vi "Read PinLevels.vi"(11 "niDigital in":refnum<class "niDigital.lvclass">) -> (2 "PinLevels":string="C:\\Sandbox\\Supporting Materials\\Digital\\Levels\\levelsheet.digilevels", 3 "niDigital out":refnum<class "niDigital.lvclass">)   [LabVIEW 2020, in "niDigital.lvclass"]
uses:
  niDigital.lvclass
  niDigital.lvclass/niDigital.ctl
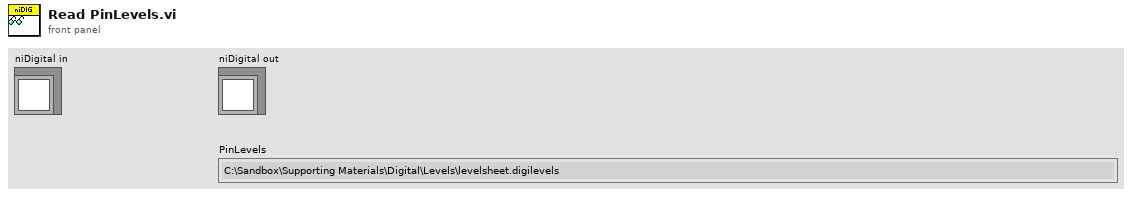
[diagram p1: front panel]
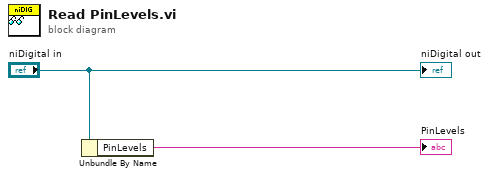
[diagram p0: block diagram]
diagram:
  n1 = Unbundle By Name("niDigital in") -> ("PinLevels"=→"PinLevels":string)
  "niDigital out" <- "niDigital in"
